vi "1_SimpleDemo_HHHisto.vi"() -> ()   [LabVIEW 2020]
uses:
  _lib/PQ/HydraHarp/HH_RefSource.ctl
  _lib/PQ/HydraHarp/HH_MeasMode.ctl
  _lib/PQ/HydraHarp/hhlib_x86_x64_UIThread.llb/HH_DllPath_global.vi
  <vilib>/Utility/error.llb/Error Cluster From Error Code.vi
  _lib/PQ/HydraHarp/HH_LibVersion_global.vi
  <vilib>/ErrorRing/Error Ring.xnode
panel:
  in  "Binning":i32(ring) caption="Resolution [ps]" items=["1", "2", "4", "8", "16", "32", "64", "128", "256", "512", "1024", "2048", "4096", "8192", "16384", "32768", "65536", "131072", "262144", "524288", "1048576", "2097152", "4194304", "8388608", "16777216", "33554432"]
  in  "HistoLength":i32(ring)=6 caption="Histo Length" items=["1024", "2048", "4096", "8192", "16384", "32768", "65536"]
  in  "Acqu.Time":i32=10000 caption="Acqu.Time [ms]" min=1 max=360000000 step=1
  in  "GlobalOffset":i32 caption="GlobalOffset [ns]" min=0 max=500000 step=1
  in  "OverflowLevel":u32=65535 min=1 step=1
  in  "StopOnOverflow":bool=TRUE
  in  "InputZeroX":i32=10 caption="ZeroCr. [mV]" min=0 max=40 step=1
  in  "InputCFDLevel":i32=50 caption="CFDLevel [mV]" min=0 max=1000 step=1
  in  "Offset":i32 caption="Offset [ps]" min=-99999 max=99999 step=1
  in  "Enable":bool=TRUE
  in  "SyncZeroX":i32=10 caption="ZeroCr. [mV]" min=0 max=40 step=1
  in  "SyncCFDLevel":i32=50 caption="CFDLevel [mV]" min=0 max=1000 step=1
  in  "SyncOffset":i32 caption="SyncOffset [ps]" min=-99999 max=99999 step=1
  in  "SyncDivider":i32(ring)=8 items=["1"=1, "2"=2, "4"=4, "8"=8, "16"=16]
  out "HistoGraph":T1(graph)={0.0, "Resolution"=0.08, "Histogram"=[]}
  out "CountRates":i32[](array[numeric]) caption="Count Rates [cps]"
  out "SyncRate":i32 caption="Sync Rate [cps]"
  in  "stop":bool
  out "error out":errorcluster
  # "Acquisition"
  # "All Channels"
  # "Sync"
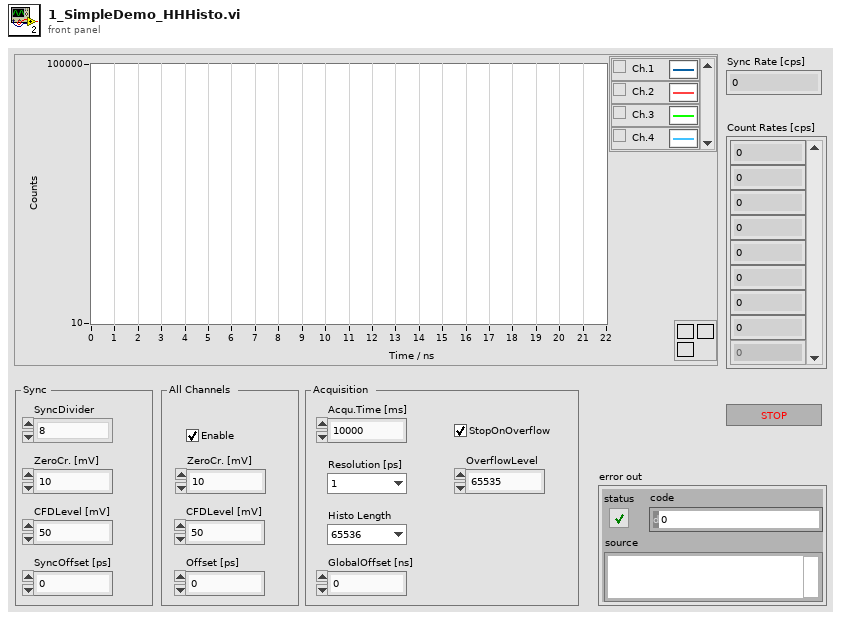
[diagram p1: front panel]
types:
  T1 = cluster{dbl, "Resolution":dbl, "Histogram":u32[][]}
  T2 = typedef "HH_MeasMode.ctl" = i32
  T3 = typedef "HH_RefSource.ctl" = enum16{"internal", "external"}
  T4 = typedef "HH_InitInfo.ctl" = cluster{"Library Version":string, "Serial No.":string, "Model":string, "Partnum":string, "Version":string, "features":i32, "nchannels":i32, "nummod":i32, "Model Codes":i32[], "Version Codes":i32[], "Base Resolution":dbl, "Bin Steps":i32}
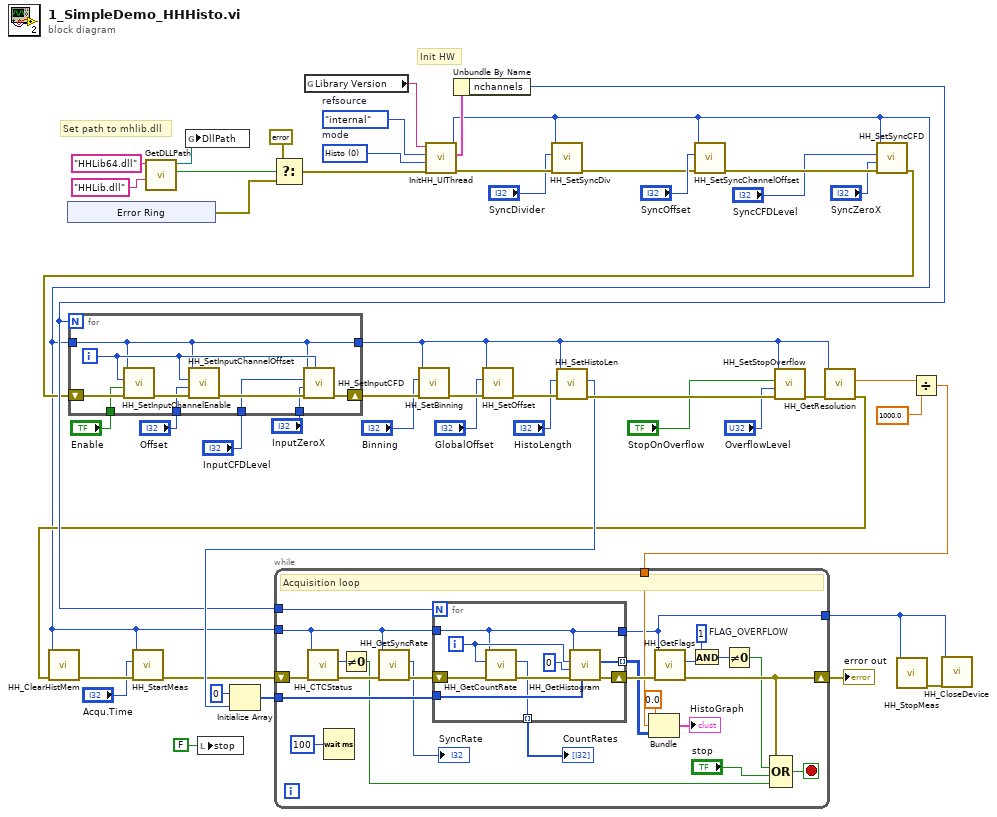
[diagram p0: block diagram]
diagram:
  w49 = T2 0 items=["Histo"=0, "T2"=2, "T3"=3, "Conti"=8]  # mode
  w50 = HH_RefSource."internal"  # refsource
  # "Init HW"
  # "Set path to mhlib.dll"
  n1 = xnode "Error Ring"() -> ("error out"=w48:errorcluster)
  n2 = call "GetDLLPath.vi"("DllName_32bit"="HHLib.dll" ("name or relative path"), "DllName_64bit"="HHLib64.dll" ("name or relative path")) -> ("file exists?"=w46:bool, "DLLPath"=w45:path)  [unwired: 8 in]
  n3 = global write "HH_DllPath_global.vi" "DllPath"(w45) -> ()
  n4 = local write "stop"(FALSE ("stop")) -> ()
  n5 = Select(t=errorcluster {"status"=FALSE, "code"=0, "source"=""} ("error IO"), s=w46, f=w48) -> (s? t:f=w42:errorcluster)
  n6 = global read "HH_LibVersion_global.vi" "Library Version"() -> (w3:string)
  n7 = call "InitHH_UIThread.vi"("error in (no error)"=w42, "mode"=w49, "refsource"=w50, "Library Version"=w3) -> ("error out"=w36:errorcluster, "Init Info"=w38:T4, "DevIdx"=w9:i32)  [unwired: 5 in]
  n8 = Unbundle By Name(w38) -> ("nchannels"=w18:i32)
  n9 = call "HH_SetSyncDiv.vi"("error in (no error)"=w36, "SyncDivider"="SyncDivider", "devidx"=w9) -> ("error out"=w35:errorcluster)  [unwired: 7 in, 1 out]
  n10 = call "HH_SetSyncChannelOffset.vi"("error in (no error)"=w35, "Offset"="SyncOffset", "devidx"=w9) -> ("error out"=w40:errorcluster)  [unwired: 7 in, 1 out]
  n11 = call "HH_SetSyncCFD.vi"("error in (no error)"=w40, "CFD ZeroCross"="SyncZeroX", "CFD Level"="SyncCFDLevel", "devidx"=w9) -> ("error out"=w17:errorcluster)  [unwired: 6 in, 1 out]
  n12 = for {
    N: w18 -> [_]
    shift-right: [w57] -> w37
    shift-left: w17 -> [w60]
    tunnel: w9 -> [w55]
    tunnel: [w55] -> w12
    tunnel: "Enable" -> [w54]
    tunnel: "Offset" -> [w53]
    tunnel: "InputZeroX" -> [w52]
    tunnel: "InputCFDLevel" -> [w51]
    i -> [w56]
    n13 = call "HH_SetInputChannelEnable.vi"("error in (no error)"=w60, "enable"=w54, "channel"=w56, "devidx"=w55) -> ("error out"=w59:errorcluster)  [unwired: 6 in, 1 out]
    n14 = call "HH_SetInputChannelOffset.vi"("error in (no error)"=w59, "Offset"=w53, "channel"=w56, "devidx"=w55) -> ("error out"=w58:errorcluster)  [unwired: 6 in, 1 out]
    n15 = call "HH_SetInputCFD.vi"("CFD Channel"=w56, "error in (no error)"=w58, "CFD ZeroCross"=w52, "CFD Level"=w51, "devidx"=w55) -> ("error out"=w57:errorcluster)  [unwired: 5 in, 1 out]
  }
  n16 = call "HH_SetBinning.vi"("error in (no error)"=w37, "Binning"="Binning", "devidx"=w12) -> ("error out"=w33:errorcluster)  [unwired: 7 in, 1 out]
  n17 = call "HH_SetOffset.vi"("error in (no error)"=w33, "Offset"="GlobalOffset", "devidx"=w12) -> ("error out"=w31:errorcluster)  [unwired: 7 in, 1 out]
  n18 = call "HH_SetHistoLen.vi"("error in (no error)"=w31, "lencode"="HistoLength", "devidx"=w12) -> ("error out"=w30:errorcluster, "actuallen"=w23:i32)  [unwired: 6 in, 1 out]
  n19 = Initialize Array(u32 0, w23) -> (w22:u32[])
  n20 = call "HH_SetStopOverflow.vi"("error in (no error)"=w30, "stopcount"="OverflowLevel", "StopOnOverflow"="StopOnOverflow", "devidx"=w12) -> ("error out"=w13:errorcluster)  [unwired: 6 in, 1 out]
  n21 = call "HH_GetResolution.vi"("error in (no error)"=w13, "devidx"=w12) -> ("error out"=w10:errorcluster, "resolution"=w11:dbl)  [unwired: 7 in, 1 out]
  n22 = call "HH_ClearHistMem.vi"("error in (no error)"=w10, "devidx"=w9) -> ("error out"=w27:errorcluster)  [unwired: 8 in, 1 out]
  n23 = call "HH_StartMeas.vi"("error in (no error)"=w27, "tacq"="Acqu.Time", "devidx"=w9) -> ("error out"=w8:errorcluster)  [unwired: 7 in, 1 out]
  n24 = Divide(x=w11, y=1000.0) -> (x/y=w19:dbl)
  n25 = while {
    shift-right: [w72] -> w25
    shift-left: w8 -> [w83]
    tunnel: w9 -> [w79]
    tunnel: w18 -> [w82]
    tunnel: w22 -> [w74]
    tunnel: w19 -> [w66]
    tunnel: [w61] -> w2
    stop <- w73 stop-if-true
    w77 = 1  # FLAG_OVERFLOW
    # "Acquisition loop"
    n26 = call "HH_CTCStatus.vi"("error in (no error)"=w83, "devidx"=w79) -> ("error out"=w81:errorcluster, "ctcstatus"=w84:i32)  [unwired: 7 in, 1 out]
    n27 = Wait (ms)(milliseconds to wait=u32 100) -> ()  [unwired: 1 out]
    n28 = Not Equal To 0?(x=w84) -> (x != 0?=w63:bool)
    n29 = call "HH_GetSyncRate.vi"("error in (no error)"=w81, "devidx"=w79) -> ("error out"=w80:errorcluster, "syncrate"=→"SyncRate":i32)  [unwired: 7 in, 1 out]
    n30 = for {
      N: w82 -> [_]
      shift-right: [w93] -> w78
      shift-left: w80 -> [w91]
      tunnel: w79 -> [w88]
      tunnel: [w88] -> w61
      tunnel: w74 -> [w87]
      tunnel: [w86] -> w69 mode=indexing
      tunnel: [w85] -> w68 mode=indexing
      i -> [w89]
      n31 = call "HH_GetCountRate.vi"("error in (no error)"=w91, "Channel"=w89, "devidx"=w88) -> ("error out"=w90:errorcluster, "rate"=w86:i32)  [unwired: 6 in, 1 out]
      n32 = call "HH_GetHistogram.vi"("Chcount"=w87, "error in (no error)"=w90, "clear"=0, "channel"=w89, "devidx"=w88) -> ("error out"=w93:errorcluster, "Histogram"=w85:u32[])  [unwired: 4 in, 1 out]
    }
    "CountRates" <- w69
    n33 = Bundle(0.0, w66, "Histogram"=w68) -> (→"HistoGraph":cluster{dbl, dbl, "Histogram":u32[][]})  [unwired: 1 in]
    n34 = call "HH_GetFlags.vi"("error in (no error)"=w78, "devidx"=w61) -> ("error out"=w72:errorcluster, "flags"=w75:i32)  [unwired: 7 in, 1 out]
    n35 = And(x=w77, y=w75) -> (x .and. y?=w76:i32)
    n36 = Not Equal To 0?(x=w76) -> (x != 0?=w71:bool)
    n37 = Compound Arithmetic op=OR(w72, w71, "stop", w63) -> (w73:bool)
  }
  "error out" <- w25
  n38 = call "HH_StopMeas.vi"("devidx"=w2) -> ("error out"=w1:errorcluster)  [unwired: 9 in, 1 out]
  n39 = call "HH_CloseDevice.vi"("error in (no error)"=w1, "devidx"=w2) -> ()  [unwired: 8 in, 2 out]
